vi "Execute.vi"(7 "Actor in":refnum<class "Actor.lvclass">, 8 "Error in":errorcluster, 11 "Stopped Msg in":refnum<class "Stopped Msg.lvclass">) -> (0 "Error out":errorcluster, 2 "Msg Output":refnum<class "Msg Output.lvclass">, 5 "Actor out":refnum<class "Actor.lvclass">)   [LabVIEW 2025, in "jettl.lvlib" / "Stopped jettl Msg.lvlib" / "Stopped Msg.lvlib" / "Stopped Msg.lvclass"]
uses:
  Stopped Msg.lvclass
  Actor/Actor.lvclass
  Msg Output/Msg Output.lvclass
  Stopped jettl Msg/Stopped jettl Msg.lvclass
  Stopped Msg.lvclass/Stopped Msg.ctl
  Stopped Msg Input/Stopped Msg Input.lvlib
  Stopped Msg Output/Stopped Msg Output.lvlib
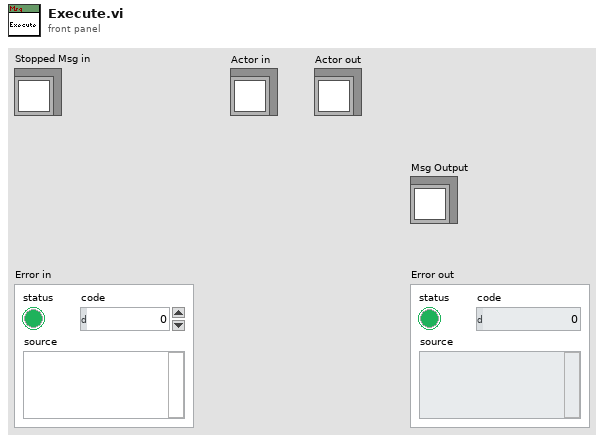
[diagram p1: front panel]
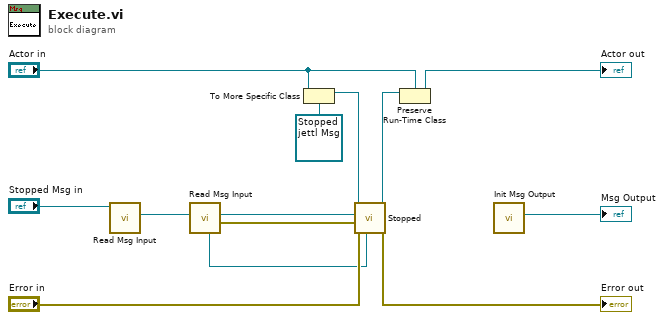
[diagram p0: block diagram]
diagram:
  n1 = call-dynamic "Read Msg Input.vi"("Stopped Msg in"="Stopped Msg in") -> ("Msg Input"=w5:refnum<class "Msg Input.lvclass">)  [unwired: 10 in]
  n2 = call "Read Msg Input.vi"("Msg Input"=w5) -> ("Error"=w1:errorcluster, "Actor"=w2:refnum<class "Actor.lvclass">, "Teller"=w4:refnum<class "Teller.lvclass">)  [unwired: 8 in]
  n3 = To More Specific Class(target class=refnum<class "Stopped jettl Msg.lvclass"> refnum ("jettl.lvlib:jettl Msg Last Ack Creator Queue.lvlib:jettl Msg Last Ack Creator Queue.lvclass"), reference="Actor in") -> (specific class reference=w8:refnum<class "Stopped jettl Msg.lvclass">)  [unwired: 1 in, 1 out]
  n4 = call-dynamic "Stopped.vi"("Teller"=w4, "Error in"="Error in", "Error"=w1, "Actor"=w2, "Stopped jettl Msg in"=w8) -> ("Error out"=→"Error out":errorcluster, "Stopped jettl Msg out"=w7:refnum<class "Stopped jettl Msg.lvclass">)  [unwired: 5 in]
  n5 = Preserve Run-Time Class(object in=w7, 2:"Actor in") -> (object out=→"Actor out":refnum<class "Actor.lvclass">)  [unwired: 1 in, 1 out]
  n6 = call "Init Msg Output.vi"() -> ("Msg Output"=→"Msg Output":refnum<class "Msg Output.lvclass">)  [unwired: 11 in]
